vi "DAQ_AO_Open.vi"(0 "reference in":refnum<class "NI_DAQ.lvclass">, 5 "error in (no error)":errorcluster) -> (14 "reference out":refnum<class "NI_DAQ.lvclass">, 19 "error out":errorcluster)   [LabVIEW 2020, in "NI_DAQ.lvclass"]
uses:
  NI_DAQ.lvclass
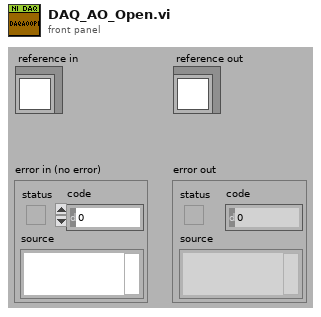
[diagram p1: front panel]
types:
  T1 = typedef "DAQ_Base.lvclass/DAQSettings.ctl" = cluster{"SampleSettings":T2, "AI_ChannelSettings":T3, "AO_ChannelSettings":T5, "Cnt_ChannelSettings":T6}
  T2 = typedef "DAQ_Base.lvclass/SampleSettings.ctl" = cluster{"samples per channel":i32, "SampleRate":dbl, "TansMaxLength":dbl, "ReadTimeOut":dbl, "时钟源":tag}
  T3 = typedef "DAQ_Base.lvclass/AI_ChannelSettings.ctl" = cluster{"AI_SettingsArry":cluster{"DeviceName":tag, "physical channels":tag, "AssignName":string, "输入信号类型":T4, "Max_value":dbl, "Min_value":dbl, "单位":i32, "shunt resistor location":i32, "external shunt resistor value":dbl, "标定系数":cluster{"Scale":dbl, "Offset":dbl}}[]}
  T4 = typedef "AI信号类型.ctl" = i32
  T5 = typedef "DAQ_Base.lvclass/AO_ChannelSettings.ctl" = cluster{"布尔":bool}
  T6 = typedef "DAQ_Base.lvclass/Cnt_ChannelSettings.ctl" = cluster{"Cnt_ChannelSettings":cluster{"类型":enum16{"Linear", "Rotate"}, "CounterNbr":tag, "AssignName":string, "单位":u16, "decoding type":u16, "PPR_DistancePerPulse":dbl, "Initial Position ":dbl, "z index enable":bool, "z index phase":i32, "source":tag}[]}
  T7 = typedef "NI_DAQ.lvclass/ObjectAttributesRef.ctl" = refnum<data-value>
  T8 = typedef "NI_DAQ.lvclass/ObjectAttributes.ctl" = cluster{"MyAttribute":dbl, "DAQ_AI_task_out":refnum<k21>, "counter_task_out":refnum<k21>[]}
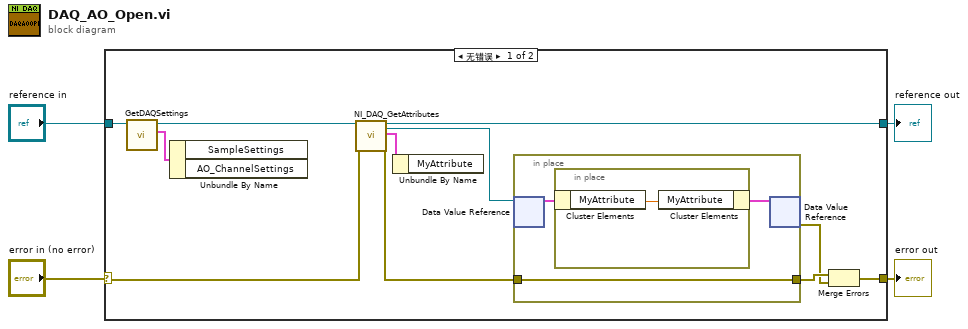
[diagram p0: block diagram]
diagram:
  n1 = case shown="无错误" "error in (no error)" {
    selector: "error in (no error)" -> [w13 w21]
    tunnel: [w15 w21] -> w3
    tunnel: [w14 w20] -> w1
    tunnel: "reference in" -> [w7 w20]
    frame No Error {
      n2 = call-dynamic "GetDAQSettings.vi"("reference in"=w7) -> ("DAQSettings"=w5:T1, "reference out"=w6:refnum<class "NI_DAQ.lvclass">)  [unwired: 8 in, 1 out]
      n3 = Unbundle By Name(w5) -> ()  [unwired: 2 out]
      n4 = call "NI_DAQ_GetAttributes.vi"("reference in"=w6, "error in (no error)"=w13) -> ("reference out"=w14:refnum<class "NI_DAQ.lvclass">, "attributes ref"=w8:T7, "attributes"=w11:T8, "error out"=w12:errorcluster)  [unwired: 14 in]
      n5 = Unbundle By Name(w11) -> ()  [unwired: 1 out]
      n6 = in-place {
        in-place-border: w12 -> [w16]
        in-place-border: [w16] -> w10
        n7 = in-place-dvr #1(w8) -> (w17:T8)  [unwired: 1 out]
        n8 = in-place {
          n9 = in-place-cluster #2(w17) -> ("MyAttribute"=w19:dbl)
          n10 = in-place-cluster #2("MyAttribute"=w19) -> (w18:T8)
        }
        n11 = in-place-dvr #1(w18) -> (w9:errorcluster)  [unwired: 1 out]
      }
      n12 = Merge Errors(w10, w9) -> (w15:errorcluster)
    }
    frame Error {
    }
  }
  "error out" <- w3
  "reference out" <- w1
